vi "To String.vi"(8 "error in (no error)":errorcluster, 11 "U32 in":refnum<class "U32.lvclass">) -> (0 "error out":errorcluster, 2 "String":string)   [LabVIEW 2020, in "Data.lvlib" / "U32.lvclass"]
doc: "Convert 'Generic Data in' to a string."
uses:
  U32.lvclass
  U32.lvclass/U32.ctl
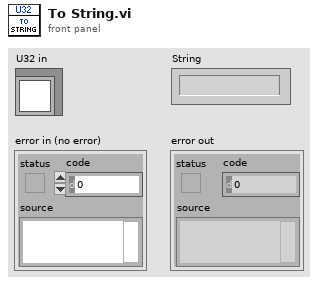
[diagram p1: front panel]
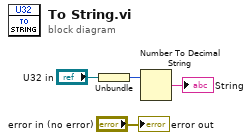
[diagram p0: block diagram]
diagram:
  n1 = Unbundle("U32 in") -> (w2:u32)
  n2 = Number To Decimal String(number=w2) -> (decimal integer string=→"String":string)  [unwired: 1 in]
  "error out" <- "error in (no error)"
